vi "GFITS_GetHdrTemplate.vi"(11 "Database RefNum":T1) -> (2 "path":path)   [LabVIEW 2016]
uses:
  DBSHAND/private/vis/DatabaseHand_RefNum.ctl
  DBSHAND/private/vis/DatabaseHand_Element_Get(path).vi
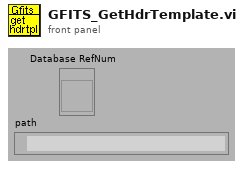
[diagram p1: front panel]
types:
  T1 = typedef "DatabaseHand_RefNum.ctl" = refnum<vi>
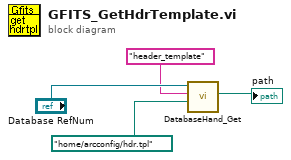
[diagram p0: block diagram]
diagram:
  n1 = call-poly "DatabaseHand_Get.vi"("default value"=path "/home/arcconfig/hdr.tpl" ("path"), "name"="header_template", "Database RefNum in"="Database RefNum") -> ("value"=→"path":path)  [unwired: 2 in, 6 out]
